vi "Set_Hi-Tec_client.vi"(5 "Row No":i32=1, 6 "Density Ratio":string="Carrier 1 only", 7 "Strength (% by volume)":dbl format="%.2f", 8 "Stack flowrate (l/min)":dbl format="%.2f", 9 "Mode":enum16{"Control Hi-Tec", "Check Hi-Tec Demands"}(ring)) -> (0 "error out":errorcluster, 1 "Flowrates (kg/min)":dbl[](array[numeric]) format="%.4f")   [LabVIEW 2010]
doc: "This is an example of using features of the VI Server as a client. It shows how you might browse from one or more applications that may be exporting data from one or more data stations. \n\nThe example shows how to query a server for its list of exported VIs, how to get references to the VIs, and how call them with the Call By Reference function."
uses:
  Anemometry/Anemometry Sub Vis/Globals/Preference_global.vi
panel:
  out "Iterations":i32
  in  "Server type":refnum<vi>
  # "-Carrier 1 only\n-Carrier 2 only\n-Enter Ratio"
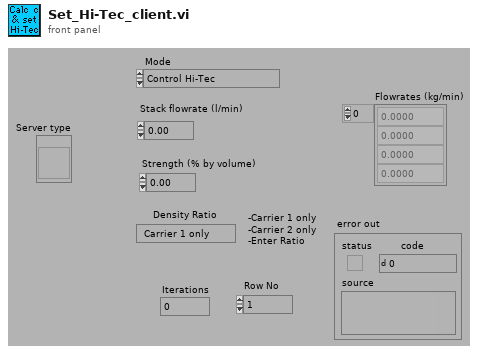
[diagram p1: front panel]
types:
  T1 = typedef "Server_Comms.ctl" = enum16{"Server Link Healthy", "Do Not Link To Server"}
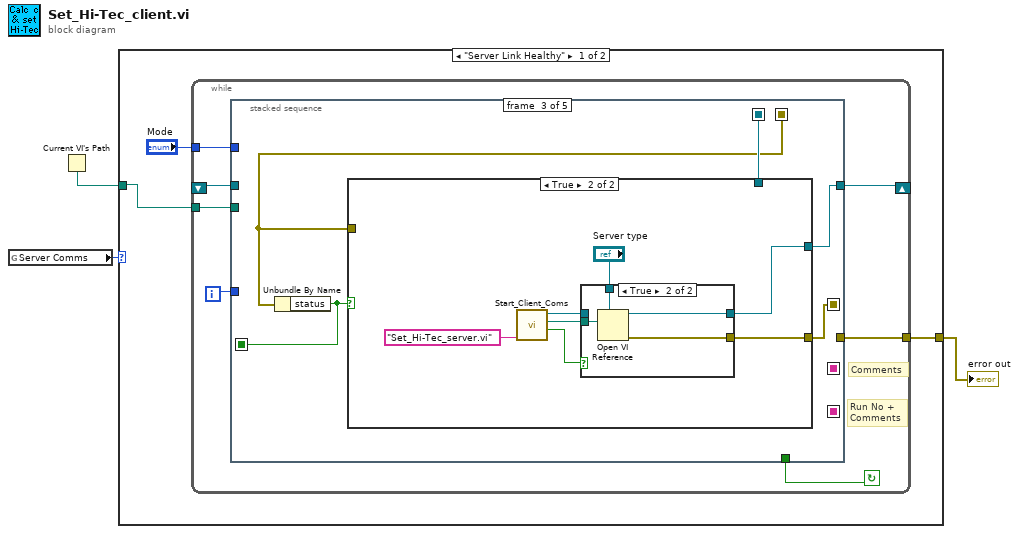
[diagram p0: block diagram]
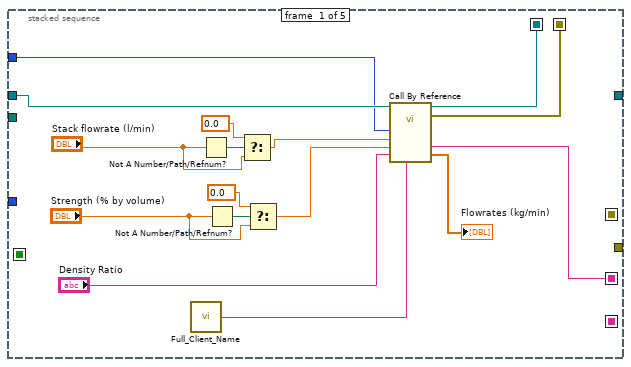
[diagram p2: hidden frame]
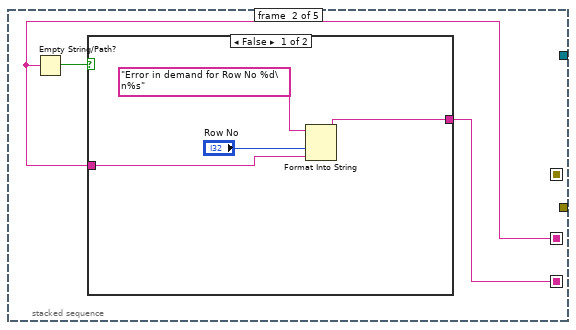
[diagram p3: hidden frame]
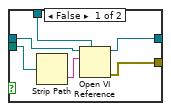
[diagram p6: hidden frame]
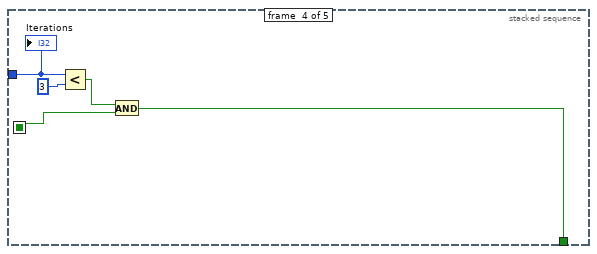
[diagram p7: hidden frame]
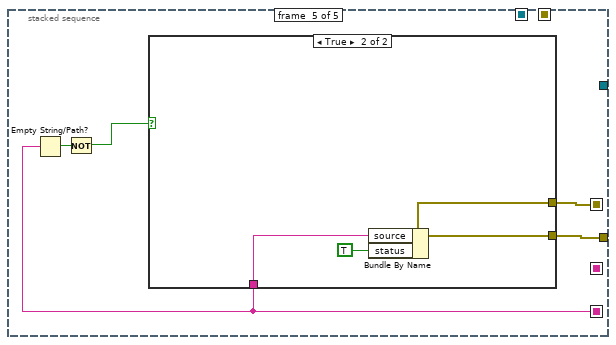
[diagram p8: hidden frame]
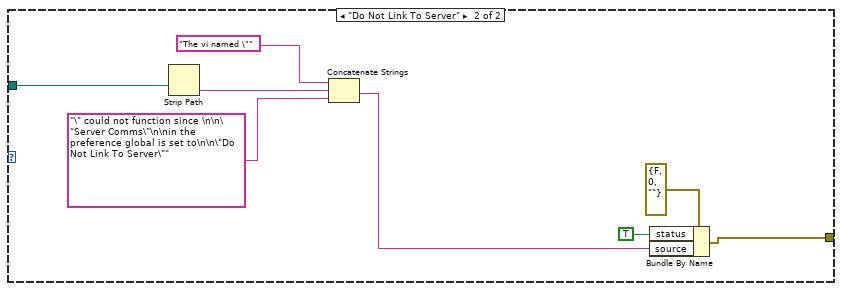
[diagram p10: hidden frame]
diagram:
  n1 = global read "Preference_global.vi" "Server Comms"() -> (w3:T1)
  n2 = Current VI's Path() -> (path=w2:path)
  n3 = case shown="\"Server Link Healthy\"" w3 {
    tunnel: [w6 w78] -> w1
    tunnel: w2 -> [w4 w77]
    frame "Server Link Healthy" {
      n4 = while {
        tunnel: w4 -> [w7]
        tunnel: "Mode" -> [w8]
        tunnel: [w9] -> w6
        shift-left: _ -> [w13]
        shift-right: [w12] -> _
        i -> [w11]
        stop <- w10 continue-if-true
        # "Run No +\nComments"
        # "Comments"
        n5 = stacked-sequence {
          seq-local: [w27 _ _ _ _] -> [_ _ w42 _ _]
          seq-local: [w26 _ _ _ _] -> [_ _ w39 _ _]
          seq-local: [_ _ w40 _ _] -> [_ _ _ w63 _]
          seq-local: [w24 _ _ _ _] -> [_ w31 _ _ _]
          seq-local: [_ w30 _ _ _] -> [_ _ _ _ w69]
          seq-local: [_ _ w38 _ _] -> [_ _ _ _ w71]
          tunnel: w13 -> [w29 _ _ _ _]
          tunnel: [_ _ w41 _ _] -> w12
          tunnel: w11 -> [_ _ _ w66 _]
          tunnel: [_ _ _ w62 _] -> w10
          tunnel: [_ _ _ _ w70] -> w9
          tunnel: w8 -> [w23 _ _ _ _]
          tunnel: w7 -> [_ _ _ _ _]
          frame #0 {
            n6 = call "Full_Client_Name.vi"() -> ("Client Name"=w22:string)
            n7 = Not A Number/Path/Refnum?(number/path/refnum="Stack flowrate (l/min)") -> (NaN/Path/Refnum?=w17:bool)
            n8 = Not A Number/Path/Refnum?(number/path/refnum="Strength (% by volume)") -> (NaN/Path/Refnum?=w21:bool)
            n9 = Select(t=0.0, s=w17, f="Stack flowrate (l/min)") -> (s? t:f=w15:dbl)
            n10 = Select(t=0.0, s=w21, f="Strength (% by volume)") -> (s? t:f=w14:dbl)
            n11 = call-by-ref "?"(reference=w29, "Client Name"=w22, "Density Ratio"="Density Ratio", "Strength (% by volume)"=w14, "Stack flowrate (l/min)"=w15, "Mode"=w23) -> (reference out=w27:refnum<vi>, error out=w26:errorcluster, "Flowrates (kg/min)"=→"Flowrates (kg/min)":dbl[], "Comment"=w24:string)  [unwired: 4 in]
          }
          frame #1 {
            n12 = Empty String/Path?(string/path=w31) -> (empty?=w32:bool)
            n13 = case shown="False" w32 {
              tunnel: w31 -> [w33 w37]
              tunnel: [w35 w37] -> w30
              frame False {
                n14 = Format Into String(format string="Error in demand for Row No %d\n%s" ("Format String"), "Row No", w33) -> (resulting string=w35:string)  [unwired: 2 in, 1 out]
              }
              frame True {
              }
            }
          }
          frame #2 {
            n15 = Unbundle By Name(w39) -> ("status"=w40:bool)
            n16 = case shown="True" w40 {
              tunnel: w42 -> [w44 _]
              tunnel: [w44 w46] -> w41
              tunnel: [w43 w45] -> w38
              tunnel: w39 -> [w43 _]
              frame False {
              }
              frame True {
                n17 = call "Start_Client_Coms.vi"("VI name to run on server"="Set_Hi-Tec_server.vi") -> ("LabVIEW application reference"=w50:refnum<vi>, "Checked VI name"=w51:path, "Local Call"=w49:bool)  [unwired: 1 in, 1 out]
                n18 = case shown="True" w49 {
                  tunnel: "Server type" -> [w53 w60]
                  tunnel: w51 -> [w54 w61]
                  tunnel: w50 -> [w52 _]
                  tunnel: [w56 w59] -> w46
                  tunnel: [w55 w58] -> w45
                  frame False {
                    n19 = Strip Path(path=w54) -> (name=w57:string)  [unwired: 1 out]
                    n20 = Open VI Reference(type specifier VI Refnum (for type only)=w53, application reference (local)=w52, vi path=w57) -> (vi reference=w56:refnum<vi>, error out=w55:errorcluster)  [unwired: 1 in, 2 out]
                  }
                  frame True {
                    n21 = Open VI Reference(type specifier VI Refnum (for type only)=w60, vi path=w61) -> (vi reference=w59:refnum<vi>, error out=w58:errorcluster)  [unwired: 1 in, 3 out]
                  }
                }
              }
            }
          }
          frame #3 {
            n22 = Less?(x=w66, y=3) -> (x < y?=w64:bool)
            n23 = And(x=w64, y=w63) -> (x .and. y?=w62:bool)
            "Iterations" <- w66
          }
          frame #4 {
            n24 = Empty String/Path?(string/path=w69) -> (empty?=w68:bool)
            n25 = Not(x=w68) -> (.not. x?=w67:bool)
            n26 = case shown="True" w67 {
              tunnel: w71 -> [w72 w76]
              tunnel: w69 -> [_ w73]
              tunnel: [w72 w75] -> w70
              frame False {
              }
              frame True {
                n27 = Bundle By Name(cluster=w76, "source"=w73, "status"=TRUE ("Bundle Element")) -> (w75:errorcluster)
              }
            }
          }
        }
      }
    }
    frame "Do Not Link To Server" {
      n28 = Strip Path(path=w77) -> (name=w83:string)  [unwired: 1 out]
      n29 = Concatenate Strings("The vi named \"", w83, "\" could not function since \n\n\"Server Comms\"\n\nin the preference global is set to\n\n\"Do Not Link To Server\"") -> (w80:string)
      n30 = Bundle By Name(cluster=errorcluster {"status"=FALSE, "code"=0, "source"=""}, "status"=TRUE ("Bundle Element"), "source"=w80) -> (w78:errorcluster)
    }
  }
  "error out" <- w1
